vi "TCL Get Fragments - 1eventNfrag.vi"(0 "event file":path, 1 "event number":i32, 3 "primary key":string, 4 "fragments":string[](array[string]), 5 "error in (no error)":errorcluster) -> (6 "fragments out":string[](array[string]), 7 "values":string[][](array[string]), 8 "error out":errorcluster)   [LabVIEW 2010]
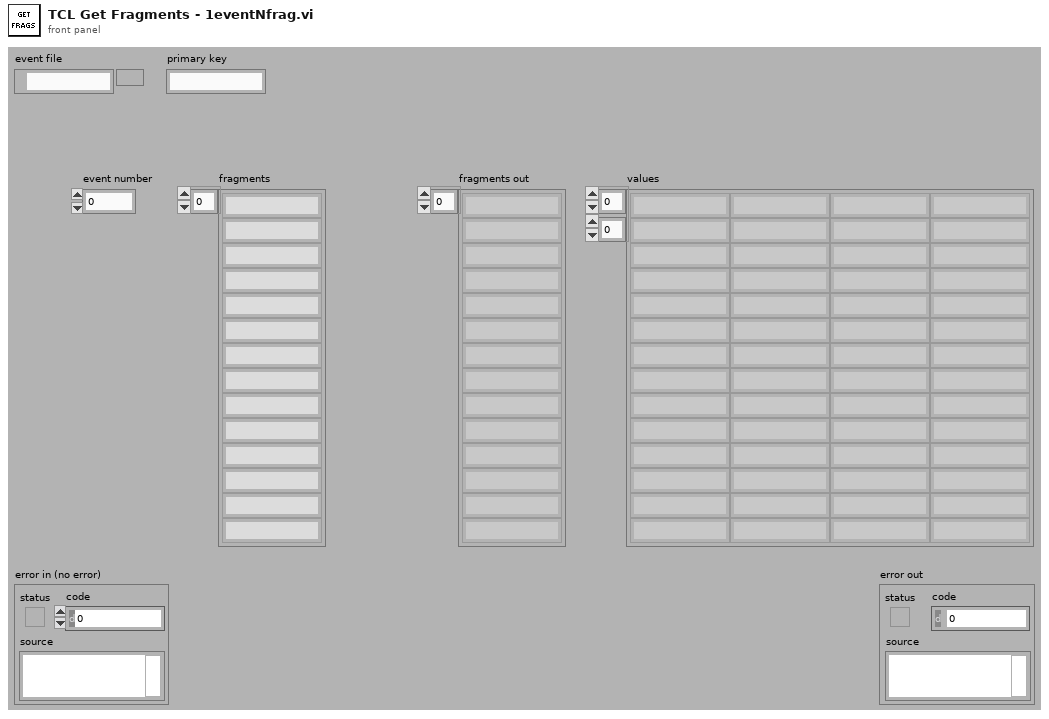
[diagram p1: front panel]
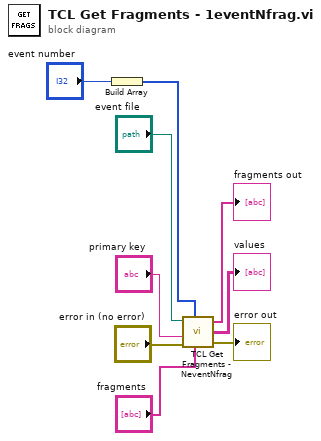
[diagram p0: block diagram]
diagram:
  n1 = Build Array("event number") -> (w3:i32[])
  n2 = call "TCL Get Fragments - NeventNfrag.vi"("event file"="event file", "event numbers"=w3, "primary key"="primary key", "fragments"="fragments", "error in (no error)"="error in (no error)") -> ("fragments out"=→"fragments out":string[], "values"=→"values":string[][], "error out"=→"error out":errorcluster)  [unwired: 1 in]
